vi "_MT_DeInit.vi"(8 "Error In":errorcluster) -> (0 "Error Out":errorcluster)   [LabVIEW 2020, in "MT_API.lvlib"]
doc: "MT_API INT32 __stdcall MT_DeInit(void);"
uses:
  MT_API.lvlib
  MT_API_64.dll
panel:
  out "函数返回值":i32
  # "释放控制设备的系统资源"
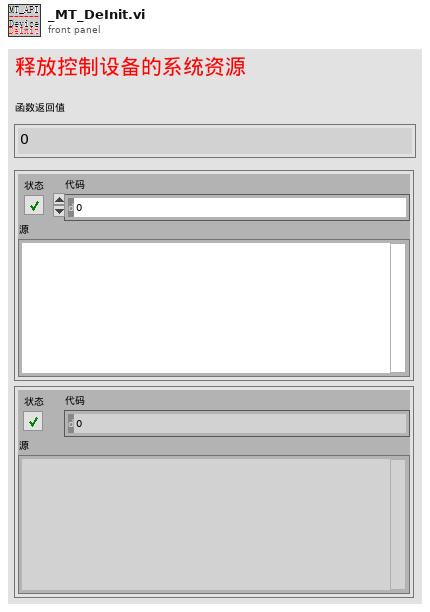
[diagram p1: front panel]
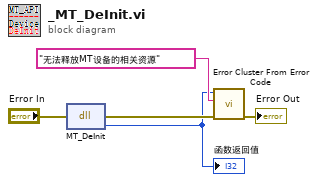
[diagram p0: block diagram]
diagram:
  n1 = dll-call lib="D:/Project NJU/lib/MT/MT_API_64.*" fn="MT_DeInit"(error in="Error In") -> (error out=w3:errorcluster, "return type"=w1:i32)  [unwired: 2 in, 1 out]
  "函数返回值" <- w1
  n2 = call <vilib>:"Error Cluster From Error Code.vi"("error in (no error)"=w3, "error message (\"\")"="无法释放MT设备的相关资源", "error code (0)"=w1) -> ("error out"=→"Error Out":errorcluster)  [unwired: 6 in]
